vi "IsConnected.vi"(8 "error in (no error)":errorcluster, 11 "BaseReader in":refnum<class "BaseReader.lvclass">) -> (0 "error out":errorcluster, 2 "connected?":bool, 3 "BaseReader out":refnum<class "BaseReader.lvclass">)   [LabVIEW 2025, in "BaseReader.lvclass"]
doc: "Returns TRUE if the Readers connection is alive"
uses:
  BaseReader.lvclass
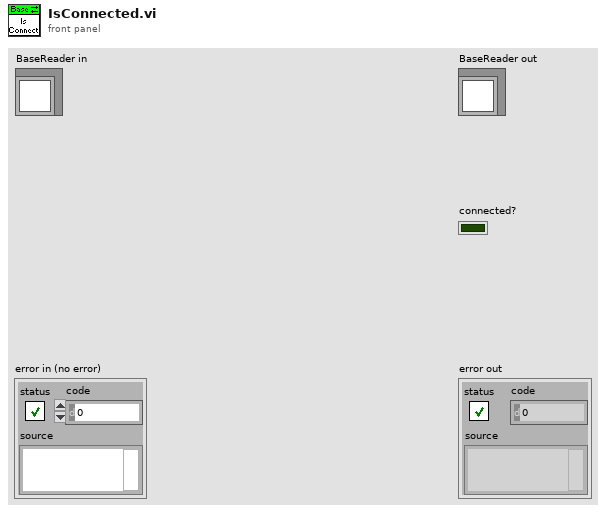
[diagram p1: front panel]
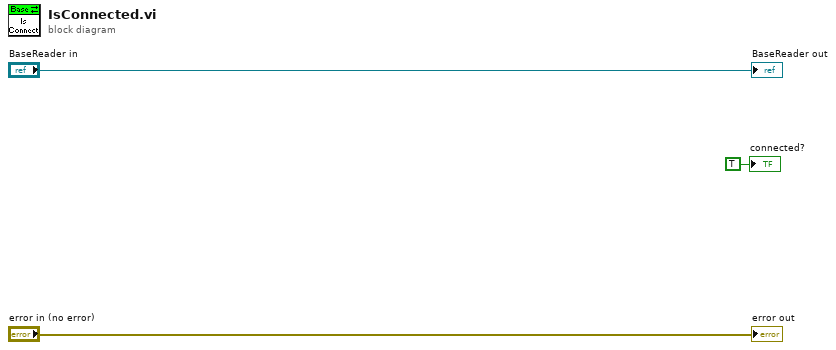
[diagram p0: block diagram]
diagram:
  "error out" <- "error in (no error)"
  "BaseReader out" <- "BaseReader in"
  "connected?" <- TRUE ("connected?")
